vi "stepper controller -- IMS -- monitor move.vi"(8 "user event":refnum<user-event>) -> ()   [LabVIEW 2018]
uses:
  stepper motor state.ctl
  stepper monitor message.ctl
  stepper motor action.ctl
panel:
  in  "stepper state":T1=enum."stopped"
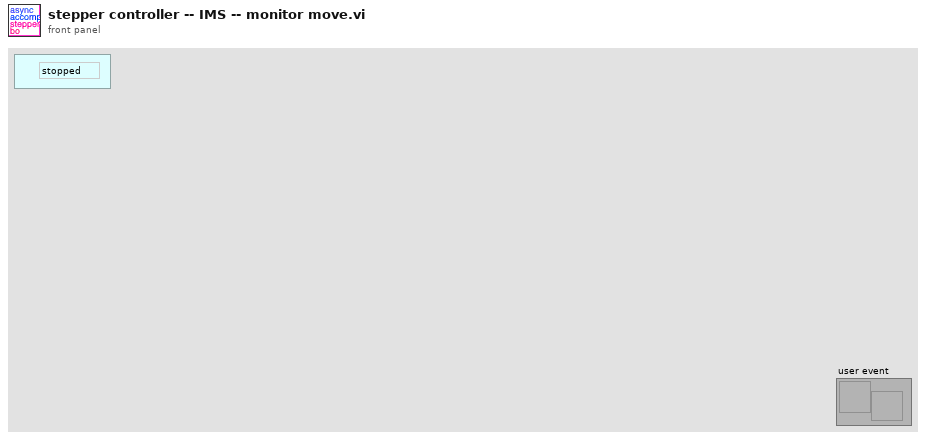
[diagram p1: front panel]
types:
  T1 = typedef "stepper motor state.ctl" = enum16{"moving", "stopped"}
  T2 = typedef "stepper monitor message.ctl" = cluster{"current position":dbl, "stepper motor state OUT":T1}
  T3 = typedef "stepper motor action.ctl" = enum16{"go", "void", "stop", "check", "init", "sync", "set", "set speed", "--check status", "--check value"}
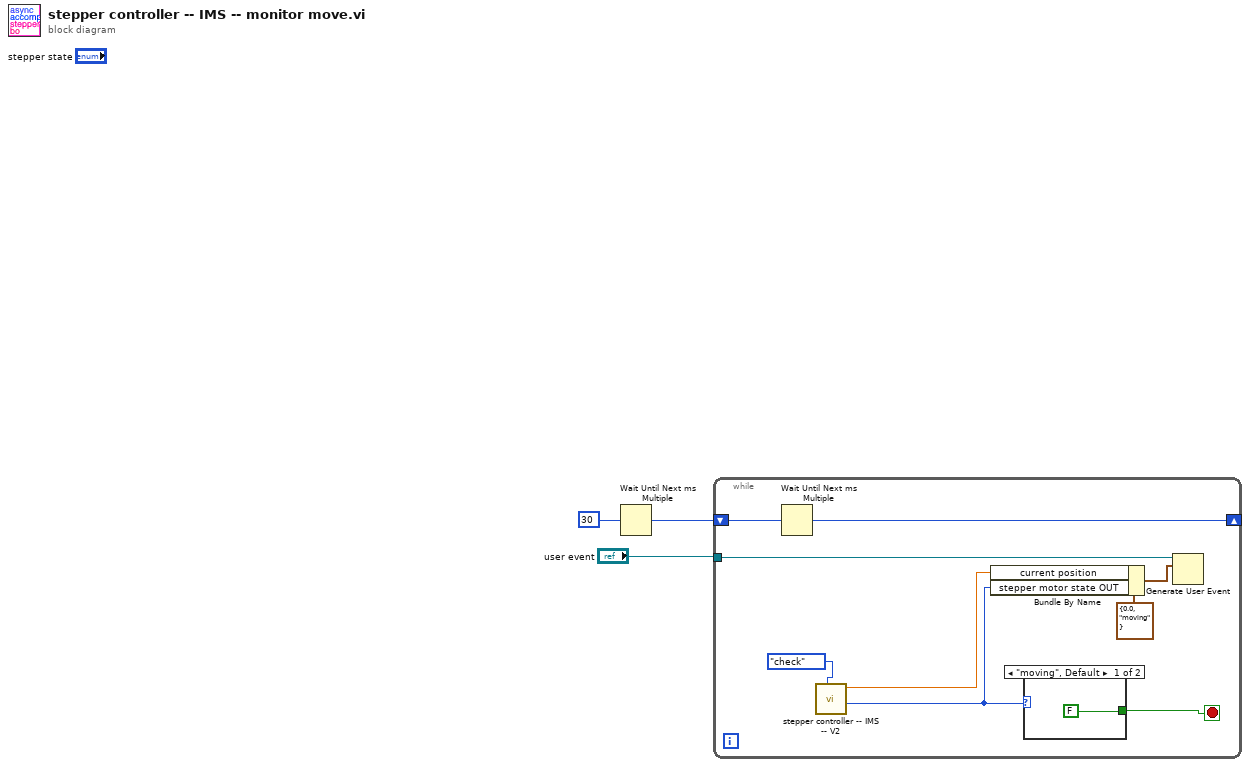
[diagram p0: block diagram]
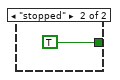
[diagram p2: hidden frame]
diagram:
  n1 = Wait Until Next ms Multiple(millisecond multiple=u32 30) -> (millisecond timer value=w1:u32)
  n2 = while {
    tunnel: "user event" -> [w12]
    shift-right: [w5] -> _
    shift-left: w1 -> [w6]
    stop <- w10 stop-if-true
    # "This loop is a consumer loop."
    n3 = Wait Until Next ms Multiple(millisecond multiple=w6) -> (millisecond timer value=w5:u32)
    n4 = call "stepper controller -- IMS -- V2.vi"("stepper driver action"=stepper_motor_action."check") -> ("stepper motor state OUT"=w4:T1, "current position"=w7:dbl)  [unwired: 8 in, 1 out]
    n5 = Bundle By Name(cluster=T2 {"current position"=0.0, "stepper motor state OUT"=enum."moving"} ("stepper monitor message"), "current position"=w7, "stepper motor state OUT"=w4) -> (w9:T2)
    n6 = case shown="\"moving\", Default" w4 {
      tunnel: [FALSE TRUE] -> w10
      frame "moving", Default {
      }
      frame "stopped" {
      }
    }
    n7 = Generate User Event(user event=w12, event data cluster=w9) -> ()  [unwired: 2 in, 2 out]
  }
